vi "Has Time Range.vi"(8 "error in (no error)":errorcluster, 9 "End":dbl, 10 "Start":dbl, 11 "Group Buffer DBL in":refnum<class "Group Buffer DBL.lvclass">) -> (0 "error out":errorcluster, 1 "Incomplete Start":dbl, 2 "Complete Range":bool, 3 "Group Buffer DBL out":refnum<class "Group Buffer DBL.lvclass">, 4 "Incomplete End":dbl)   [LabVIEW 2020, in "VolatusHistorian.lvlib" / "Group Buffer DBL.lvclass"]
uses:
  Group Buffer DBL.lvclass
  Group Buffer DBL.lvclass/Group Buffer DBL.ctl
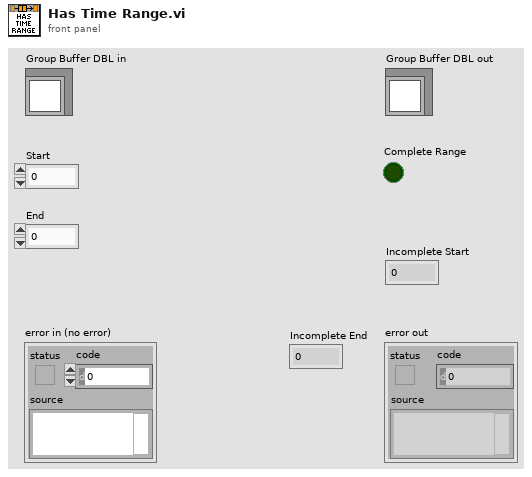
[diagram p1: front panel]
types:
  T1 = typedef "VolatusHistorian.lvlib/Group Buffer DBL.lvclass/Ref.ctl" = cluster{"Time":refnum<queue>, "Channel Name Map":map{string, i32}, "Group Info":T2, "Channels":refnum<class "Channel Buffer DBL.lvclass">[], "Channel Names":string[]}
  T2 = typedef "VectoConfig.lvlib/Group Info.ctl" = cluster{"System":string, "Cluster":string, "Node":string, "Task":string, "Name":string}
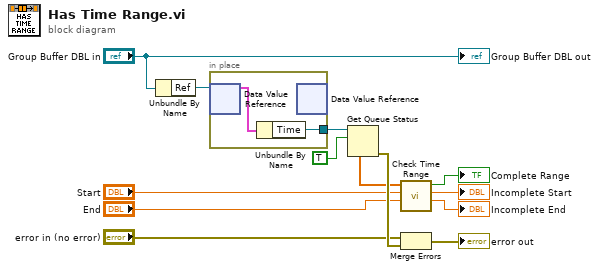
[diagram p0: block diagram]
diagram:
  n1 = Unbundle By Name("Group Buffer DBL in") -> ("Ref"=w11:refnum<data-value>)
  n2 = in-place {
    in-place-border: [w14] -> w9
    n3 = in-place-dvr #1(w11) -> (w15:T1)  [unwired: 1 out]
    n4 = Unbundle By Name(w15) -> ("Time"=w14:refnum<queue>)
    n5 = in-place-dvr #1() -> ()  [unwired: 1 in, 2 out]
  }
  n6 = Get Queue Status(queue=w9, return elements? (F)=TRUE) -> (error out=w13:errorcluster, elements=w7:dbl[])  [unwired: 1 in, 6 out]
  n7 = call "Check Time Range.vi"("End"="End", "Start"="Start", "Time"=w7) -> ("Incomplete End"=→"Incomplete End":dbl, "Incomplete Start"=→"Incomplete Start":dbl, "Complete Range"=→"Complete Range":bool)  [unwired: 6 in]
  n8 = Merge Errors("error in (no error)", w13) -> (→"error out":errorcluster)
  "Group Buffer DBL out" <- "Group Buffer DBL in"
